vi "filter.wait.for.command.vi"(11 "filter.data in":T1 {"get.state"."v"."Quantity" format="%.0x"; "get.state"."v"."OrderId" format="%.0x"; "mem.cmd"."ord.2"."v"."Quantity" format="%016x"; "mem.cmd"."ord.2"."v"."OrderId" format="%016x"; "mem.cmd"."ord.1"."v"."Quantity" format="%016x"; "mem.cmd"."ord.1"."v"."OrderId" format="%016x"; "mem.cmd"."ticker"."v"."Symbol" format="%016x"; "mem.cmd"."order.slot.value"."Quantity" format="%016x"; "mem.cmd"."order.slot.value"."OrderId" format="%016x"; "debug"."v"."slot.3" format="%.0x"; "debug"."v"."slot.2" format="%.0x"; "debug"."v"."slot.1" format="%.0x"; "debug"."v"."slot.0" format="%.0x"; "Scratch"."OrderId" format="%016x"; "hash.2"."data.in" format="%.0x"; "hash.2"."crc32.out" format="%.0x"; "hash.1"."data.in" format="%.0x"; "hash.1"."crc32.out" format="%.0x"}) -> (2 "Ready.for.OrderBook.Command.Input":bool, 3 "filter.data out":T1 {"get.state"."v"."Quantity" format="%.0x"; "get.state"."v"."OrderId" format="%.0x"; "mem.cmd"."ord.2"."v"."Quantity" format="%016x"; "mem.cmd"."ord.2"."v"."OrderId" format="%016x"; "mem.cmd"."ord.1"."v"."Quantity" format="%016x"; "mem.cmd"."ord.1"."v"."OrderId" format="%016x"; "mem.cmd"."ticker"."v"."Symbol" format="%016x"; "mem.cmd"."order.slot.value"."Quantity" format="%016x"; "mem.cmd"."order.slot.value"."OrderId" format="%016x"; "debug"."v"."slot.3" format="%.0x"; "debug"."v"."slot.2" format="%.0x"; "debug"."v"."slot.1" format="%.0x"; "debug"."v"."slot.0" format="%.0x"; "Scratch"."OrderId" format="%016x"; "hash.2"."data.in" format="%.0x"; "hash.2"."crc32.out" format="%.0x"; "hash.1"."data.in" format="%.0x"; "hash.1"."crc32.out" format="%.0x"})   [LabVIEW 2020]
uses:
  <vilib>/rvi/DataTransferAndStorage/Container/XNode/niFpgaContainer.xnode
  filter.states.ctl
  order.slot.ctl
  ticker.slot.ctl
  filter.memory.command.ctl
  filter.debug.slot.ctl
  filter.debug.ctl
  Market.Data.Common/fpga/orderbook.command.ctl
  Market.Data.Common/fpga/fpganow.common.fpga.lvlib
  Market.Data.Common/fpga/orderbook.command.type.ctl
  order.slot.hm.ctl
  order.slot.access.ctl
  ticker.slot.access.ctl
  <vilib>/rvi/FIFO/Fifo_Resource/nirvififoEmulationRead.vi
  filter.data.scratch.ctl
  filter.data.ctl
  filter.state.slot.ctl
  filter.state.ctl
  filter.hash.ctl
  Filter.lvclass
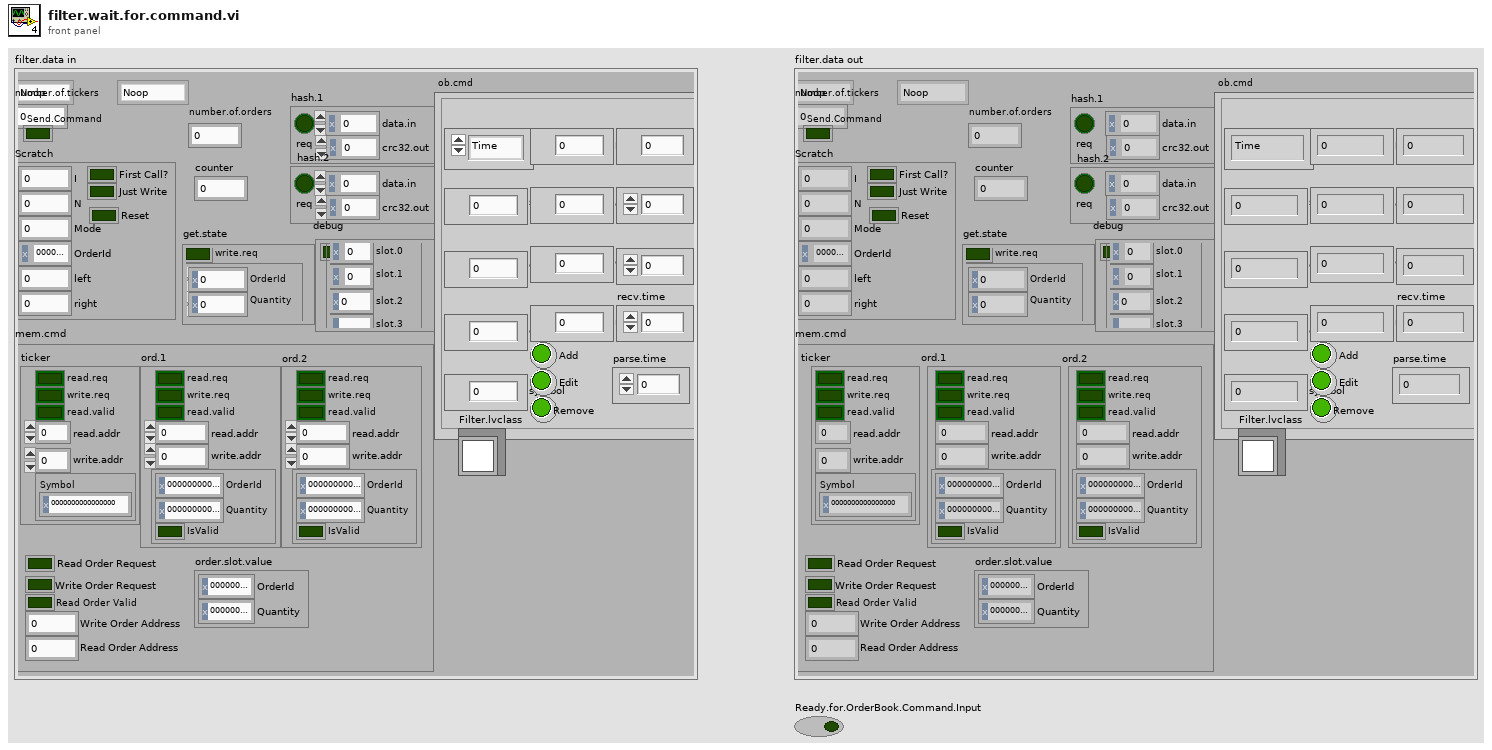
[diagram p1: front panel]
types:
  T1 = typedef "filter.data.ctl" = cluster{"filter.state":T2, "number.of.tickers":u32, "filter.saved.state":T2, "Send.Command":bool, "hash.1":T3, "hash.2":T3, "Scratch":T4, "debug":T5, "mem.cmd":T7, "get.state":T13, "ob.cmd":T15, "number.of.orders":u32, "Filter.lvclass":refnum<class "Filter.lvclass">, "counter":i16}
  T2 = typedef "filter.states.ctl" = enum16{"Noop", "Reset", "Debug", "Configuration", "Wait.for.Command", "Filter.Add", "Filter.Other", "Insert.Order", "Delete Order", "Get.State", "Get.Watchlist", "Get.Memory"}
  T3 = typedef "filter.hash.ctl" = cluster{"req":bool, "data.in":u64, "crc32.out":u32}
  T4 = typedef "filter.data.scratch.ctl" = cluster{"I":u32, "N":u32, "Mode":u32, "OrderId":u64, "First Call?":bool, "Just Write":bool, "left":u32, "right":u32, "Reset":bool}
  T5 = typedef "filter.debug.ctl" = cluster{"write":bool, "v":T6}
  T6 = typedef "filter.debug.slot.ctl" = cluster{"slot.0":u64, "slot.1":u64, "slot.2":u64, "slot.3":u64}
  T7 = typedef "filter.memory.command.ctl" = cluster{"Read Order Request":bool, "Write Order Request":bool, "Read Order Valid":bool, "Write Order Address":u32, "Read Order Address":u32, "order.slot.value":T8, "ticker":T9, "ord.1":T11, "ord.2":T11}
  T8 = typedef "order.slot.ctl" = cluster{"OrderId":u64, "Quantity":u64}
  T9 = typedef "ticker.slot.access.ctl" = cluster{"read.req":bool, "write.req":bool, "read.valid":bool, "read.addr":u32, "write.addr":u32, "v":T10}
  T10 = typedef "ticker.slot.ctl" = cluster{"Symbol":u64}
  T11 = typedef "order.slot.access.ctl" = cluster{"read.req":bool, "write.req":bool, "read.valid":bool, "read.addr":u32, "write.addr":u32, "v":T12}
  T12 = typedef "order.slot.hm.ctl" = cluster{"OrderId":u64, "Quantity":u64, "IsValid":bool}
  T13 = typedef "filter.state.ctl" = cluster{"write.req":bool, "v":T14}
  T14 = typedef "filter.state.slot.ctl" = cluster{"OrderId":u64, "Quantity":u64}
  T15 = typedef "fpganow.common.fpga.lvlib/orderbook.command.ctl" = cluster{"type":T16, "side":u8, "orderId ":u64, "quantity":u32, "symbol":u64, "price":u64, "executed.qty":u32, "canceled.qty":u32, "remaining.qty":u32, "seconds":u64, "nanoseconds":u64, "Add":bool, "Edit":bool, "Remove":bool, "seq no":u32, "recv.time":u64, "parse.time":u64}
  T16 = typedef "fpganow.common.fpga.lvlib/orderbook.command.type.ctl" = enum8{"Time", "AddOrder", "OrderExecuted", "OrderExecutedAtPrice", "ReduceSize", "ModifyOrder", "DeleteOrder", "Get.Everything", "Get.All.Orders", "Get.Top"}
  T17 = cluster{"type":enum8{"Time", "AddOrder", "OrderExecuted", "OrderExecutedAtPrice", "ReduceSize", "ModifyOrder", "DeleteOrder", "Get.Everything", "Get.All.Orders", "Get.Top"}, "side":u8, "orderId ":u64, "quantity":u32, "symbol":u64, "price":u64, "executed.qty":u32, "canceled.qty":u32, "remaining.qty":u32, "seconds":u64, "nanoseconds":u64, "Add":bool, "Edit":bool, "Remove":bool, "seq no":u32}
  T18 = enum8{"Time", "AddOrder", "OrderExecuted", "OrderExecutedAtPrice", "ReduceSize", "ModifyOrder", "DeleteOrder", "Get.Everything", "Get.All.Orders", "Get.Top"}
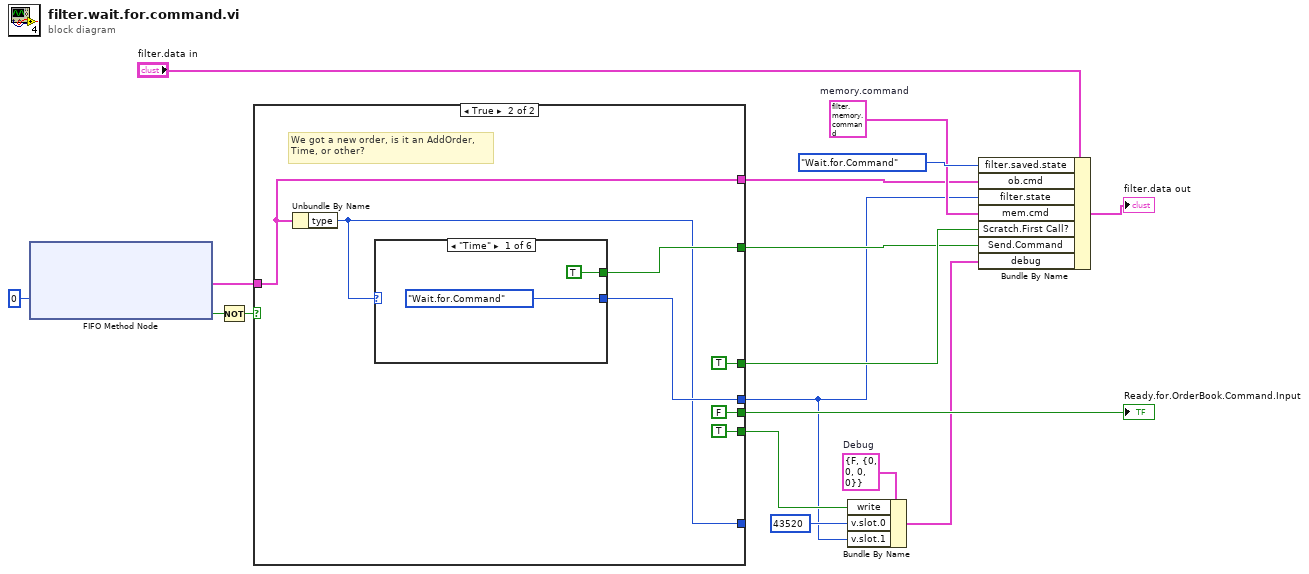
[diagram p0: block diagram]
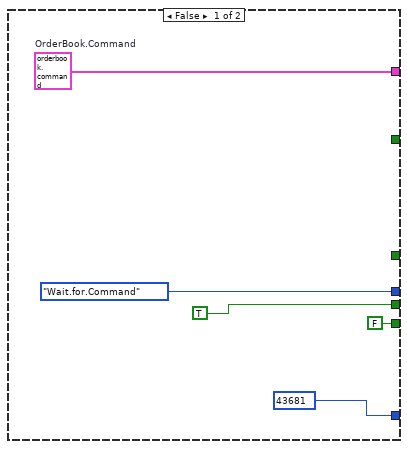
[diagram p2: hidden frame]
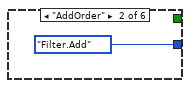
[diagram p3: hidden frame]
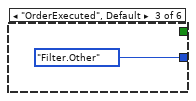
[diagram p4: hidden frame]
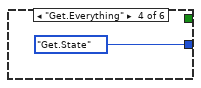
[diagram p5: hidden frame]
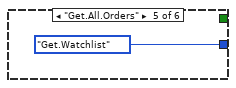
[diagram p6: hidden frame]
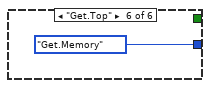
[diagram p7: hidden frame]
diagram:
  w13 = T5 {"write"=FALSE, "v"={"slot.0"=0, "slot.1"=0, "slot.2"=0, "slot.3"=0}}  # Debug
  w12 = T7 {"Read Order Request"=FALSE, "Write Order Request"=FALSE, "Read Order Valid"=FALSE, "Write Order Address"=0, "Read Order Address"=0, "order.slot.value"={"OrderId"=0, "Quantity"=0}, "ticker"={"read.req"=FALSE, "write.req"=FALSE, "read.valid"=FALSE, "read.addr"=0, "write.addr"=0, "v"={"Symbol"=0}}, "ord.1"={"read.req"=FALSE, "write.req"=FALSE, "read.valid"=FALSE, "read.addr"=0, "write.addr"=0, "v"={"OrderId"=0, "Quantity"=0, "IsValid"=FALSE}}, "ord.2"={"read.req"=FALSE, "write.req"=FALSE, "read.valid"=FALSE, "read.addr"=0, "write.addr"=0, "v"={"OrderId"=0, "Quantity"=0, "IsValid"=FALSE}}}  # memory.command
  n1 = xnode ("FIFO Method Node")("Timeout"=0) -> ("Element"=w8:T17, "Timed Out?"=w7:bool)  [unwired: 1 in, 1 out]
  n2 = Not(x=w7) -> (.not. x?=w9:bool)
  n3 = case shown="True" w9 {
    tunnel: w8 -> [_ w29]
    tunnel: [w20 w29] -> w10
    tunnel: [filter.states."Wait.for.Command" ("filter.state") w25] -> w1
    tunnel: [TRUE FALSE] -> w11
    tunnel: [FALSE TRUE] -> w16
    tunnel: [u64 43681 ("OrderId") w23] -> _
    tunnel: [_ TRUE ("First Call?")] -> w17
    tunnel: [_ w24] -> w3
    frame False {
      w20 = T15 {"type"=enum."AddOrder", "side"=0, "orderId "=0, "quantity"=0, "symbol"=0, "price"=0, "executed.qty"=0, "canceled.qty"=0, "remaining.qty"=0, "seconds"=0, "nanoseconds"=0, "Add"=FALSE, "Edit"=FALSE, "Remove"=FALSE, "seq no"=0, "recv.time"=0, "parse.time"=0}  # OrderBook.Command
    }
    frame True {
      # "We got a new order, is it an AddOrder,\nTime, or other?"
      n4 = Unbundle By Name(w29) -> ("type"=w23:T18)
      n5 = case shown="\"Time\"" w23 {
        tunnel: [filter.states."Wait.for.Command" ("t") filter.states."Filter.Add" ("t") filter.states."Filter.Other" ("t") filter.states."Get.State" ("t") filter.states."Get.Watchlist" ("t") filter.states."Get.Memory" ("t")] -> w25
        tunnel: [TRUE _ _ _ _ _] -> w24
        frame "Time" {
        }
        frame "AddOrder" {
        }
        frame "OrderExecuted", Default {
        }
        frame "Get.Everything" {
        }
        frame "Get.All.Orders" {
        }
        frame "Get.Top" {
        }
      }
    }
  }
  "Ready.for.OrderBook.Command.Input" <- w11
  n6 = Bundle By Name(cluster=w13, "write"=w16, "v.slot.0"=u64 43520 ("OrderId"), "v.slot.1"=w1) -> (w4:T5)
  n7 = Bundle By Name(cluster="filter.data in", "filter.saved.state"=filter.states."Wait.for.Command", "ob.cmd"=w10, "filter.state"=w1, "mem.cmd"=w12, "Scratch.First Call?"=w17, "Send.Command"=w3, "debug"=w4) -> (→"filter.data out":T1)
